vi "Handle.vi"(7 "Event Actor in":refnum<class "Event Actor.lvclass">, 11 "Error Event State in":refnum<class "Error Event State.lvclass">) -> (2 "Destroy?":bool, 5 "Event Actor out":refnum<class "Event Actor.lvclass">)   [LabVIEW 2021, in "jettl.lvlib" / "Error Event State.lvclass"]
uses:
  Error Event State.lvclass
  Event Actor/Event Actor.lvclass
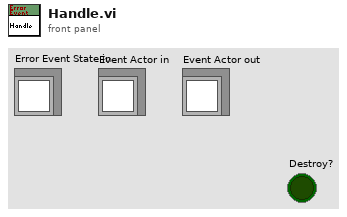
[diagram p1: front panel]
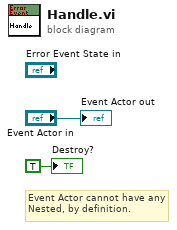
[diagram p0: block diagram]
diagram:
  # "Event Actor cannot have any Nested, by definition."
  "Destroy?" <- TRUE ("Destroy?")
  "Event Actor out" <- "Event Actor in"
